vi "master command fg.vi"(1 "Loop Progress":u8, 2 "Menu":T1) -> (0 "Loop Progress":u8)   [LabVIEW 2013]
uses:
  typedefs/fg_typedef.ctl
panel:
  # "This FG writes the command it was given most recently"
  # "Then when cancel is called, the cancel state machine adapts to cancel the most recent command"
  # "This excludes shooting and passing"
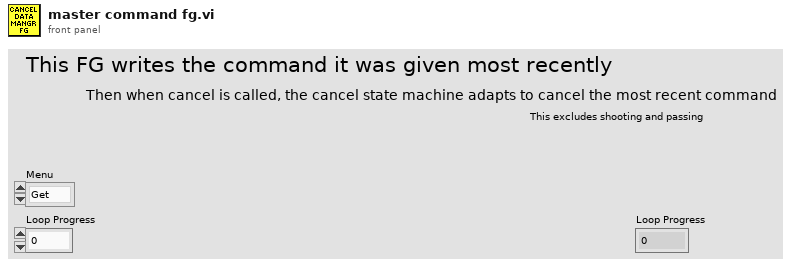
[diagram p1: front panel]
types:
  T1 = typedef "fg_typedef.ctl" = enum16{"Get", "Set"}
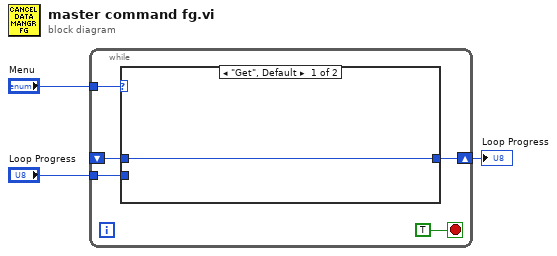
[diagram p0: block diagram]
diagram:
  n1 = while {
    tunnel: "Loop Progress" -> [w6]
    tunnel: "Menu" -> [w7]
    shift-right: [w5] -> w1
    shift-left: _ -> [w4]
    stop <- TRUE stop-if-true
    n2 = case shown="\"Get\", Default" w7 {
      tunnel: w6 -> [_ w10]
      tunnel: [w9 w10] -> w5
      tunnel: w4 -> [w9 _]
      frame "Get", Default {
      }
      frame "Set" {
      }
    }
  }
  "Loop Progress" <- w1
